vi "niP2P Merge Errors.vi"(0 "error code":i32, 5 "stream handle (0)":u32, 11 "error in":errorcluster) -> (15 "error out":errorcluster)   [LabVIEW 2010]
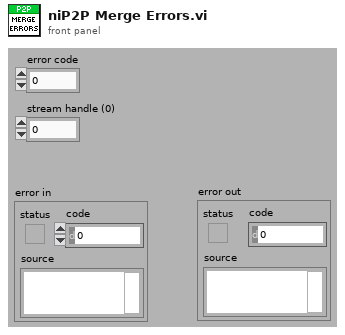
[diagram p1: front panel]
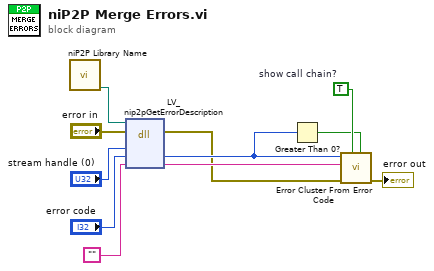
[diagram p0: block diagram]
diagram:
  w7 = TRUE  # show call chain?
  n1 = call <vilib>:"niP2P Library Name.vi"() -> ("nip2p libname"=w2:path)  [unwired: 10 in]
  n2 = dll-call lib="?" fn="LV_nip2pGetErrorDescription"(path in=w2, error in="error in", "streamHandle"="stream handle (0)", "errorCode"="error code", "errorText"="") -> (error out=w1:errorcluster, "errorCode"=w4:i32, "errorText"=w6:string)  [unwired: 3 in, 1 out]
  n3 = Greater Than 0?(x=w4) -> (x > 0?=w3:bool)
  n4 = call <vilib>:"Error Cluster From Error Code.vi"("is warning? (False)"=w3, "show call chain? (False)"=w7, "error in (no error)"=w1, "error message (\"\")"=w6, "error code (0)"=w4) -> ("error out"=→"error out":errorcluster)  [unwired: 4 in]
